vi "VI-Typedef To Table.vi"(0 "Path to typdef":path, 11 "error in (no error)":errorcluster) -> (4 "Table":T1[](array[typedef]), 15 "error out":errorcluster)   [LabVIEW 2020]
uses:
  VI-Typedef Table Element.ctl
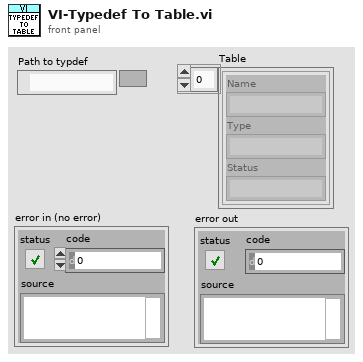
[diagram p1: front panel]
types:
  T1 = typedef "VI-Typedef Table Element.ctl" = cluster{"Name":string, "Type":string, "Status":string}
  T2 = typedef "LVNumericRepresentation.ctl" = enum32{"Extended Precision", "Double Precision", "Single Precision", "Long", "Word", "Byte", "Unsigned Long", "Unsigned Word", "Unsigned Byte", "Complex Extended", "Complex Double", "Complex Single", "Quad", "Unsigned Quad", "Fixed-Point"}
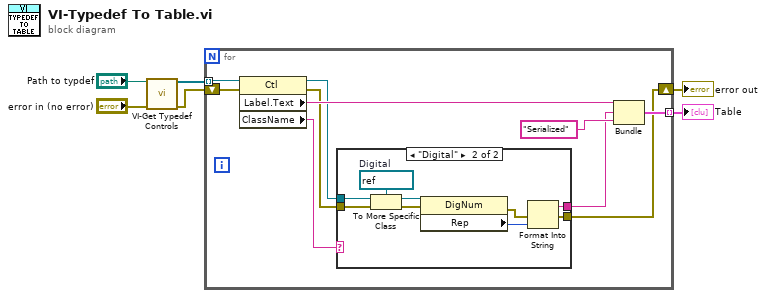
[diagram p0: block diagram]
diagram:
  n1 = call "VI-Get Typedef Controls.vi"("Path to typdef"="Path to typdef", "error in (no error)"="error in (no error)") -> ("Controls[]"=w5:refnum<vi>[], "error out"=w2:errorcluster)  [unwired: 12 in]
  n2 = for {
    tunnel: w5 -> [w16] mode=indexing
    tunnel: [w14] -> w6 mode=indexing
    shift-right: [w8] -> w1
    shift-left: w2 -> [w12]
    n3 = property class="Ctl"(reference=w16, error in=w12) -> (reference out=w9:refnum<vi>, error out=w10:errorcluster, "Label.Text"=w15:string, "ClassName"=w11:string)
    n4 = case shown="\"Digital\"" w11 {
      selector: w11 -> [w17 _]
      tunnel: w10 -> [w18 w25]
      tunnel: w9 -> [_ w26]
      tunnel: [w18 w20] -> w8
      tunnel: [w17 w19] -> w7
      frame "False", Default {
      }
      frame "Digital" {
        w27 = refnum<vi> refnum  # Digital
        n5 = To More Specific Class(target class=w27, reference=w26, error in=w25) -> (specific class reference=w24:refnum<vi>, error out=w23:errorcluster)
        n6 = property class="DigNum"(reference=w24, error in=w23) -> (error out=w22:errorcluster, "Rep"=w21:T2)  [unwired: 1 out]
        n7 = Format Into String(error in=w22, w21) -> (resulting string=w19:string, error out=w20:errorcluster)  [unwired: 2 in]
      }
    }
    n8 = Bundle("Label.Text"=w15, w7, "Serialized") -> (w14:cluster{"Label.Text":string, string, string})  [unwired: 1 in]
  }
  "Table" <- w6
  "error out" <- w1
